vi "MGC_SendCommand.vi"(8 "Error in":errorcluster, 10 "Command":string="idn?", 11 "Device":refnum<k24>) -> (0 "Error out":errorcluster, 2 "Answer":string, 3 "Device":refnum<k24>)   [LabVIEW 2016]
doc: "Sends a command to the device and returns its answer.\n\nCommand: Command to send to the device (see manual of the device for details)\nAnswer: Answer of the device according to sent command"
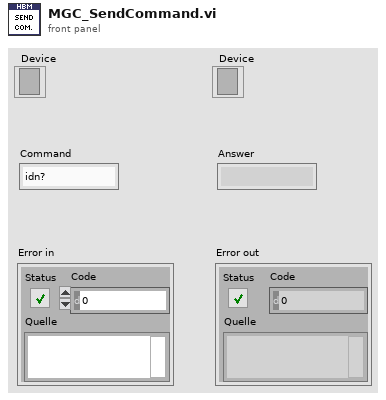
[diagram p1: front panel]
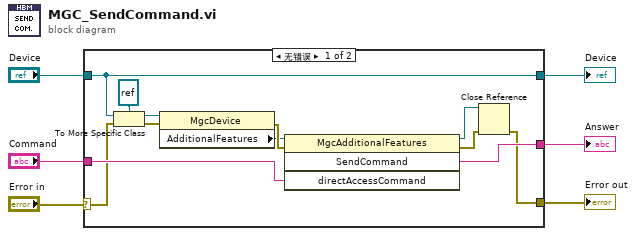
[diagram p0: block diagram]
diagram:
  n1 = case shown="无错误" "Error in" {
    selector: "Error in" -> [w9 w20]
    tunnel: "Device" -> [w18 w19]
    tunnel: [w18 w19] -> w5
    tunnel: [w12 w20] -> w3
    tunnel: "Command" -> [w16 _]
    tunnel: [w15 _] -> w1
    frame No Error {
      n2 = To More Specific Class(target class=refnum<k24> refnum ("Zielklasse"), reference=w18, error in=w9) -> (specific class reference=w17:refnum<k24>, error out=w14:errorcluster)
      n3 = property on="Eigenschaftsknoten" class="MgcDevice"(reference=w17, error in=w14) -> (error out=w13:errorcluster, "AdditionalFeatures"=w7:refnum<k24>)  [unwired: 1 out]
      n4 = invoke on="Methodenknoten" class="MgcAdditionalFeatures" method="SendCommand"(reference=w7, error in=w13, "directAccessCommand"=w16) -> (reference out=w10:refnum<k24>, error out=w11:errorcluster, "SendCommand"=w15:string)  [unwired: 1 in, 1 out]
      n5 = Close Reference(reference=w10, error in (no error)=w11) -> (error out=w12:errorcluster)
    }
    frame Error {
    }
  }
  "Error out" <- w3
  "Device" <- w5
  "Answer" <- w1
